vi "ErrorLookup.vi"(1 "Error Code":i32 min=-8 max=0 step=1) -> (0 "Error":string)   [LabVIEW 2012]
panel:
  # "This example serves to translate error codes into a \nshort readable form.  It can be used as a SubVI to aid\nin debugging."
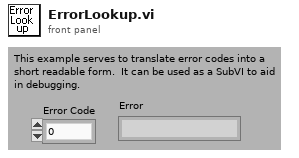
[diagram p1: front panel]
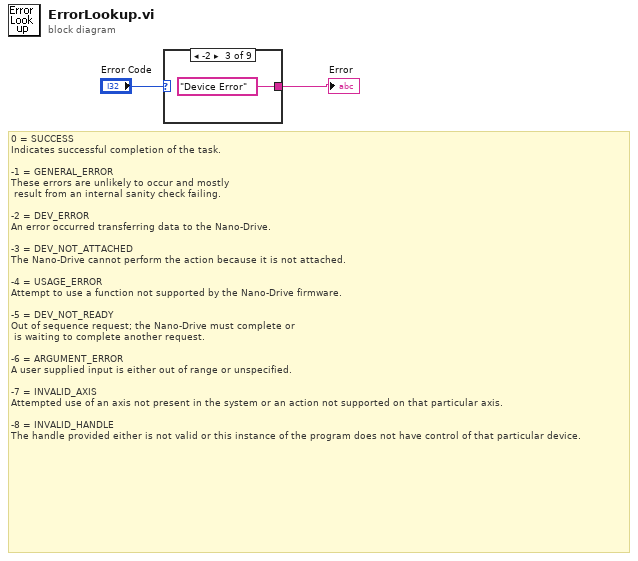
[diagram p0: block diagram]
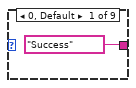
[diagram p2: hidden frame]
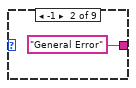
[diagram p3: hidden frame]
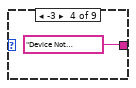
[diagram p4: hidden frame]
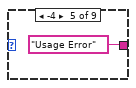
[diagram p5: hidden frame]
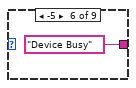
[diagram p6: hidden frame]
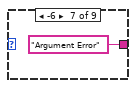
[diagram p7: hidden frame]
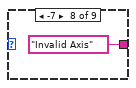
[diagram p8: hidden frame]
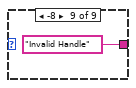
[diagram p9: hidden frame]
diagram:
  # "0 = SUCCESS\nIndicates successful completion of the task.\n\n-1 = GENERAL_ERROR \nThese errors are unlikely to occur and mostly \n\tresult from an internal sanity check failing.\n\n-2 = DEV_ERROR\nAn error occurred transferring data to the Nano-Drive.\n\n-3 = DEV_NOT_ATTACHED\nThe Nano-Drive cannot perform the action because it is not attached.\n\n-4 = USAGE_ERROR\nAttempt to use a function not supported by the Nano-Drive firmware.\n\n-5 = DEV_NOT_READY\nOut of sequence request; the Nano-Drive must complete or\n\tis waiting to complete another request.\n\n-6 = ARGUMENT_ERROR  \nA user supplied input is either out of range or unspecified.\n\n-7 = INVALID_AXIS \nAttempted use of an axis not present\tin the system or an action not supported on that particular axis.\n\n-8 = INVALID_HANDLE\nThe handle provided either is not valid or this instance of the program does not have control of that particular device."
  n1 = case shown="-2" "Error Code" {
    tunnel: ["Success" "General Error" "Device Error" "Device Not Attached" "Usage Error" "Device Busy" "Argument Error" "Invalid Axis" "Invalid Handle"] -> w1
    frame 0, Default {
    }
    frame -1 {
    }
    frame -2 {
    }
    frame -3 {
    }
    frame -4 {
    }
    frame -5 {
    }
    frame -6 {
    }
    frame -7 {
    }
    frame -8 {
    }
  }
  "Error" <- w1
